vi "GetStartPoint.vi"(8 "error in (no error)":errorcluster, 11 "reference in":refnum<class "Row.lvclass">) -> (0 "error out":errorcluster, 2 "StartPoint":T1, 3 "reference in":refnum<class "Row.lvclass">)   [LabVIEW 2012, in "Row.lvclass"]
uses:
  Row.lvclass
  Glyph_class/Position.ctl
  Glyph_class/Glyph.lvclass
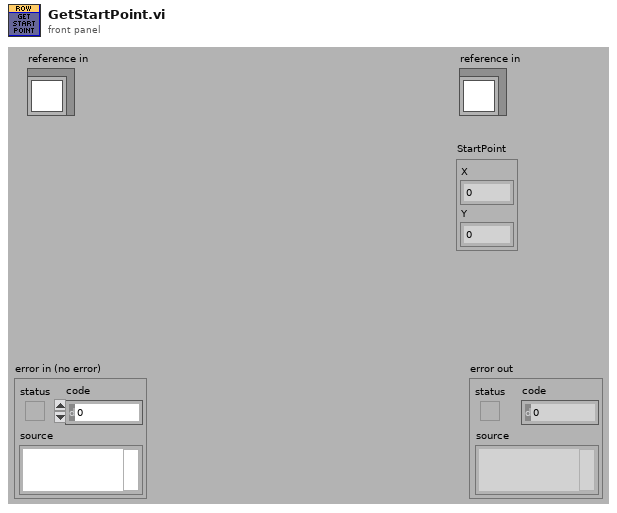
[diagram p1: front panel]
types:
  T1 = typedef "Glyph.lvclass/Position.ctl" = cluster{"X":i32, "Y":i32}
  T2 = typedef "Row.lvclass/ObjectAttributes.ctl" = cluster{"Characters":refnum<class "Character.lvclass">[], "StartPoint":T1, "CharacterSpacing":i32}
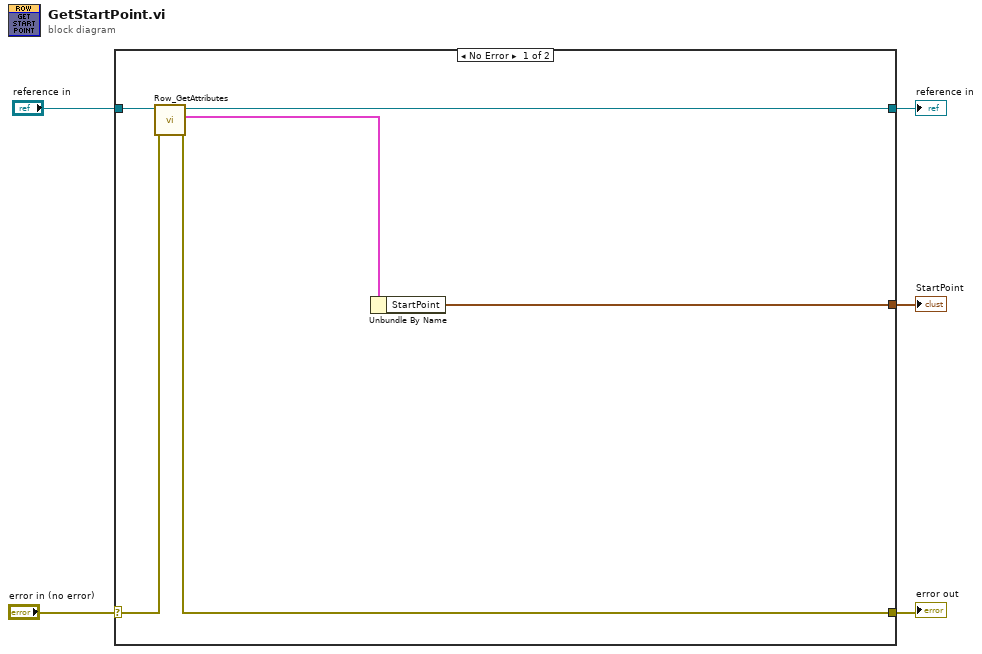
[diagram p0: block diagram]
diagram:
  n1 = case shown="No Error" "error in (no error)" {
    selector: "error in (no error)" -> [w11 w13]
    tunnel: [w9 w13] -> w4
    tunnel: [w7 w12] -> w2
    tunnel: "reference in" -> [w8 w12]
    tunnel: [w6 _] -> w1
    frame No Error {
      n2 = call "Row_GetAttributes.vi"("error in (no error)"=w11, "reference in"=w8) -> ("error out"=w9:errorcluster, "Data"=w10:T2, "reference out"=w7:refnum<class "Row.lvclass">)  [unwired: 6 in, 1 out]
      n3 = Unbundle By Name(w10) -> ("StartPoint"=w6:T1)
    }
    frame Error {
    }
  }
  "error out" <- w4
  "reference in" <- w2
  "StartPoint" <- w1
